vi "Sonar_MLS.vi"() -> ()   [LabVIEW 2016]
uses:
  <vilib>/rvi/Analysis/host/Private/Sample Rate To Loop Time (ticks).vi
  <vilib>/FPGAPlugInAG/sbRIO-9633/niLvFpga_Open_sbRIO-9633.vi
  <vilib>/rvi/interface/common/dynamic/niFpgaDynamicAddResources.vi
  <vilib>/Utility/error.llb/Error Cluster From Error Code.vi
  <vilib>/rvi/errors/niLvFpgaAdjustHostInterfaceError.vi
  <vilib>/FPGAPlugInAG/Dynamic/niLvFpga_Run_Dynamic.vi
  <vilib>/Utility/file.llb/Write Delimited Spreadsheet (string).vi
  <vilib>/FPGAPlugInAG/Dynamic/niLvFpga_Close_Dynamic.vi
  <vilib>/rvi/interface/nirviOpenFPGA/nirviOpenFPGA.xnode
  FPGA Bitfiles/sbRIOtest_FPGATarget2_DAQgenV4_wkZzV3iQ7fI.lvbitx
  DAQgenV4.vi
  <vilib>/rvi/interface/nirviReadWriteControl/nirviReadWriteControl.xnode
  <vilib>/rvi/interface/nirviMethod/nirviMethod.xnode
  <vilib>/rvi/interface/nirviCloseFPGA/nirviCloseFPGA.xnode
  <vilib>/rvi/errors/niLvFpgaMergeErrorWithErrorCode.vi
  <vilib>/rvi/interface/Simulation/niFpgaSimulationCallBeginRW.vi
  <vilib>/FPGAPlugInAG/Dynamic/niLvFpga_StartFifo_Dynamic.vi
  <vilib>/rvi/Analysis/host/Public/NI_FpgaMspHost.lvlib
  NiFpgaLv.dll
  <vilib>/FPGAPlugInAG/Dynamic/niLvFpga_ReadFifo_Dynamic.vi
  <vilib>/FPGAPlugInAG/Dynamic/niLvFpga_WriteFifo_Dynamic.vi
panel:
  out "Fs, out (Hz)":dbl format="%#_6p"
  out "Fs, in (Hz)":dbl
  in  "Iterations":i32=25
  in  "VISA resource name":refnum<visa-resource-name>="ASRL1::INSTR"
  out "?":string
  in  "Interpulse Time (ms)":u32=1300
  out "Aggregate Input Rate (Hz)":dbl
  in  "?":bool
  in  "Chirp Length (ms)":i32=5
  out "Echo":dbl[][](graph)
  in  "Samples to Read":i32=4000
  out "Wave Output":dbl[](graph)=[0.5, 0.5001220703125, 0.50048828125, 0.5010986328125, 0.501953125, 0.5029296875, 0.504150390625, 0.50537109375, 0.5064697265625, 0.50732421875, 0.5078125, 0.50732421875, 0.505859375, 0.5030517578125, 0.4986572265625, 0.4925537109375, 0.48486328125, 0.47607421875, 0.466796875, 0.4583740234375, 0.4522705078125, 0.4501953125, 0.4539794921875, 0.4647216796875, 0.4830322265625, 0.5078125, 0.5364990234375, 0.564697265625, 0.5865478515625, 0.5960693359375, 0.5880126953125, 0.56005859375, 0.51416015625, 0.4578857421875, 0.4039306640625, 0.3671875, 0.362060546875, 0.395751953125, 0.46533203125, 0.55419921875, 0.6357421875, 0.6796875, 0.6634521484375, 0.5838623046875, 0.463134765625, 0.345458984375, 0.2823486328125, 0.309814453125, 0.4273681640625, 0.5899658203125, 0.7216796875, 0.750244140625, 0.647705078125, 0.455810546875, 0.2747802734375, 0.213623046875, 0.32275390625, 0.5509033203125, 0.760986328125, 0.8094482421875, 0.6470947265625, 0.3704833984375, 0.1728515625, 0.2109375, 0.4754638671875, 0.7733154296875, 0.862060546875, 0.650146484375, 0.298583984375, 0.10986328125, 0.26806640625, 0.6494140625, 0.9031982421875, 0.7716064453125, 0.362548828125, 0.0799560546875, 0.2296142578125, 0.675048828125, 0.94189453125, 0.7196044921875, 0.238525390625, 0.0513916015625, 0.3975830078125, 0.877685546875, 0.8968505859375, 0.410400390625, 0.0303955078125, 0.2659912109375, 0.822265625, 0.94384765625, 0.4442138671875, 0.0172119140625, 0.28759765625, 0.8759765625, 0.9034423828125, 0.3118896484375, 0.0091552734375, 0.483642578125, 0.9871826171875, 0.6937255859375, 0.076171875, 0.17529296875, 0.8331298828125, 0.90869140625, 0.259033203125, 0.044921875, 0.663330078125, 0.975830078125, 0.391357421875, 0.0184326171875, 0.5802001953125, 0.979248046875, 0.4212646484375, 0.0286865234375, 0.6031494140625, 0.9560546875, 0.348388671875, 0.072509765625, 0.71923828125, 0.8770751953125, 0.2025146484375, 0.2047119140625, 0.87158203125, 0.6761474609375, 0.0802001953125, 0.477783203125, 0.9163818359375, 0.351318359375, 0.1612548828125, 0.8004150390625, 0.6805419921875, 0.1173095703125, 0.532958984375, 0.8494873046875, 0.2613525390625, 0.312255859375, 0.8492431640625, 0.446044921875, 0.2041015625, 0.7640380859375, 0.5853271484375, 0.1837158203125, 0.6695556640625, 0.660888671875, 0.2047119140625, 0.603271484375, 0.686279296875, 0.2335205078125, 0.573974609375, 0.6785888671875, 0.2564697265625, 0.5772705078125, 0.6473388671875, 0.274658203125, 0.603515625, 0.595458984375, 0.2991943359375, 0.6385498046875, 0.52490234375, 0.344482421875, 0.6614990234375, 0.446533203125, 0.4193115234375, 0.648193359375, 0.385986328125, 0.5128173828125, 0.5849609375, 0.37744140625, 0.587158203125, 0.4908447265625, 0.43603515625, 0.595458984375, 0.42333984375, 0.524658203125, 0.53076171875, 0.435302734375, 0.566650390625, 0.458251953125, 0.5052490234375, 0.52685546875, 0.4564208984375, 0.5426025390625, 0.471923828125, 0.5081787109375, 0.509765625, 0.479248046875, 0.5234375, 0.4805908203125, 0.51171875, 0.4964599609375, 0.4971923828125, 0.50634765625, 0.492919921875, 0.5059814453125, 0.4959716796875, 0.5020751953125, 0.499267578125, 0.5, 0.5001220703125, 0.4998779296875]
  in  "Initial Frequency (Hz)":dbl=20000.0
  in  "Final Frequency (Hz)":dbl=100000.0
  in  "Amplitude":dbl=2.0
  # "Echo-Pulse Sonar V6"
  # "To access the data, go to your web browser and type ftp://169.254.32.143/ni-rt/startup/"
  # "Wave Maker"
  # "Adding:\n-Digital signal trigger outputs to Pi\n-Sending data via serial to the Pi"
  # "Logger"
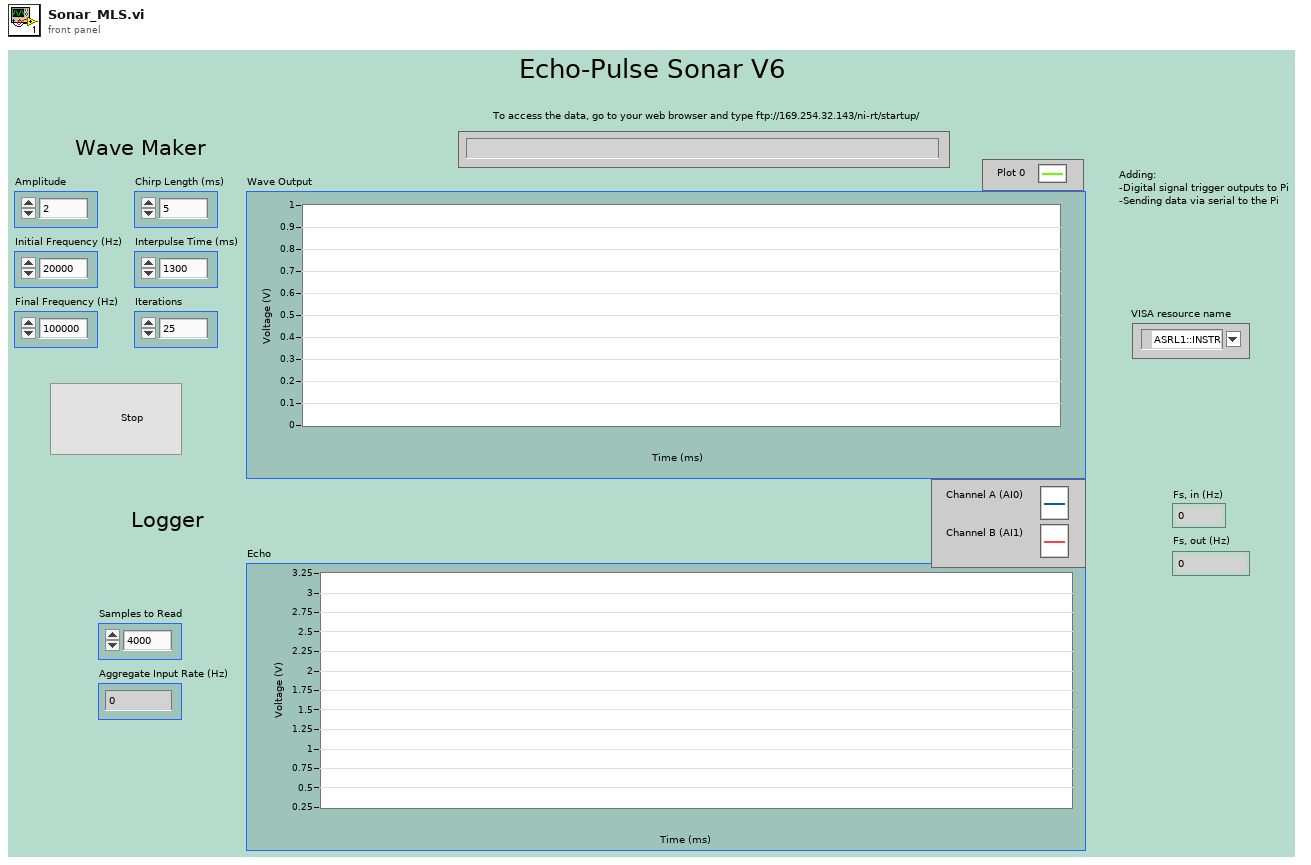
[diagram p1: front panel]
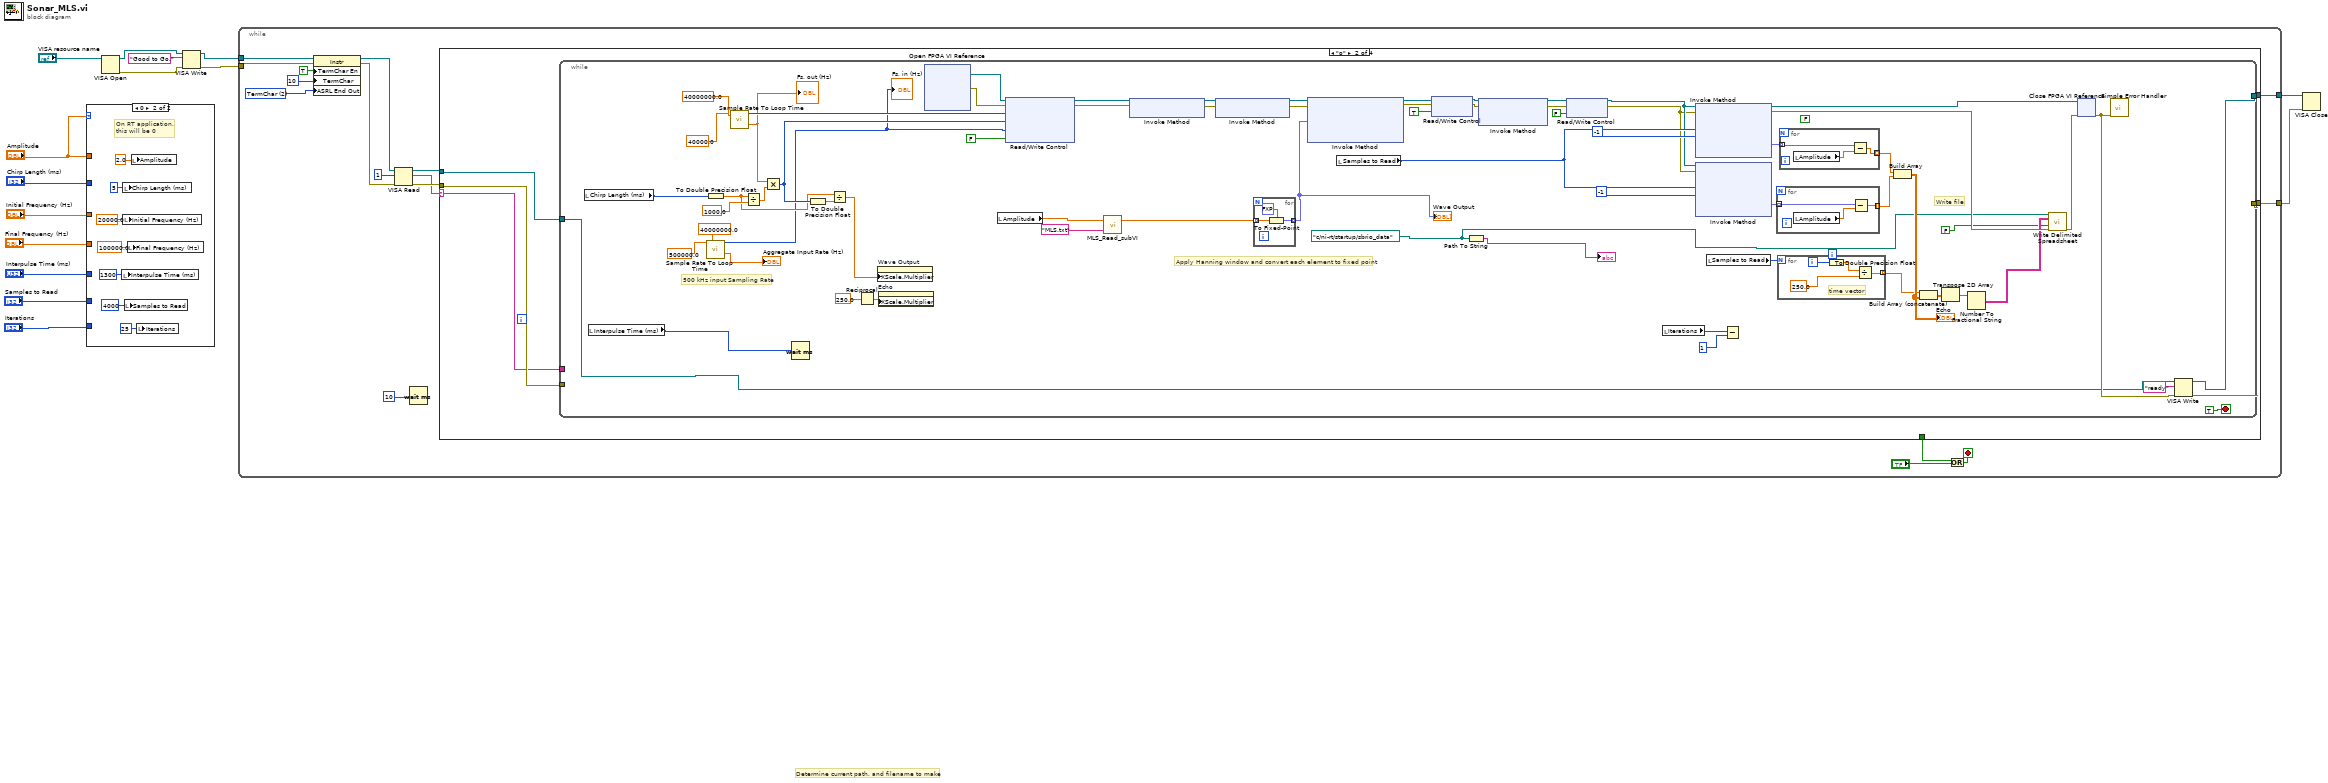
[diagram p0: block diagram]
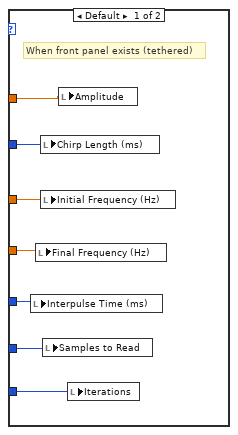
[diagram p2: hidden frame]
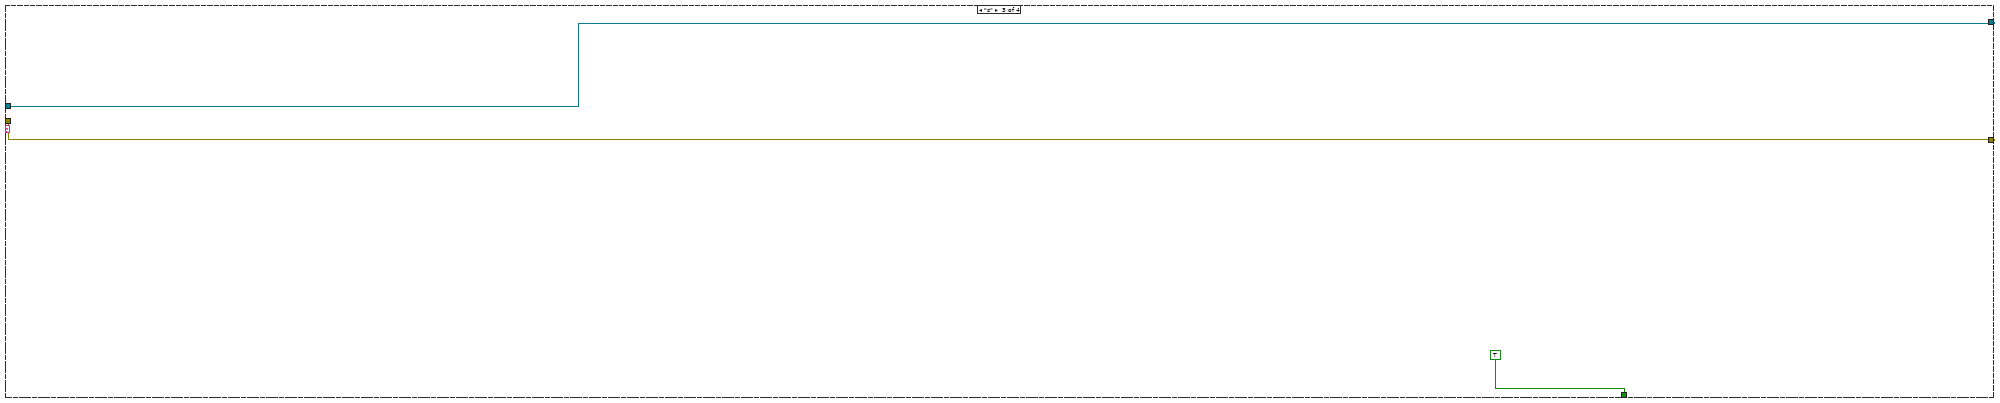
[diagram p4: hidden frame]
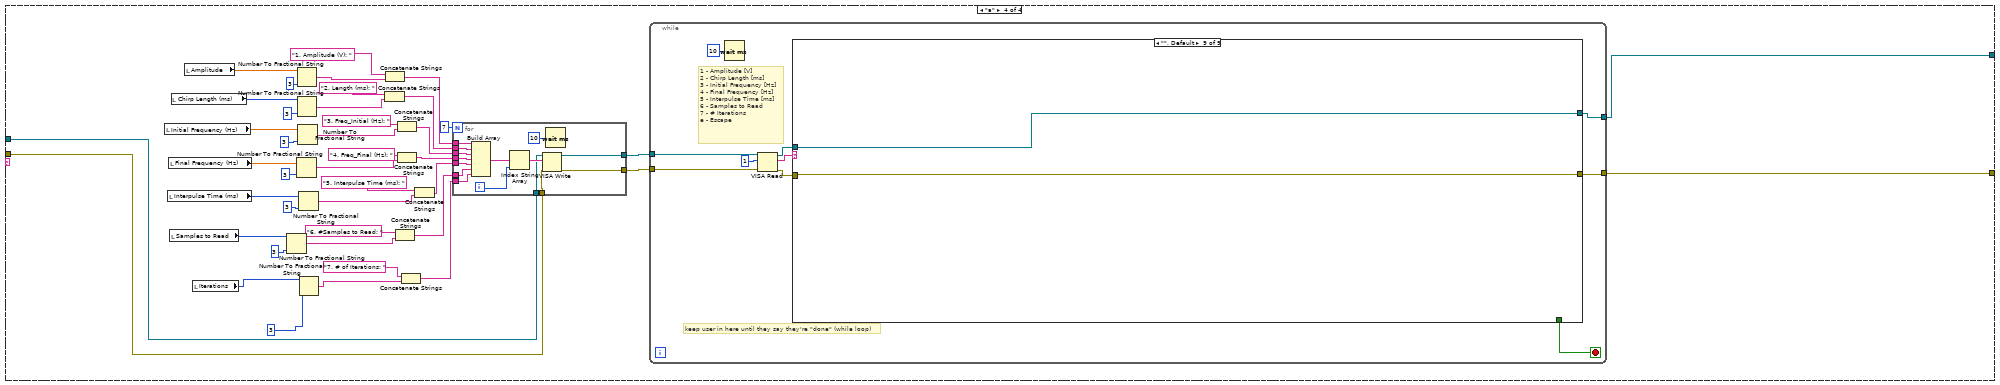
[diagram p5: hidden frame]
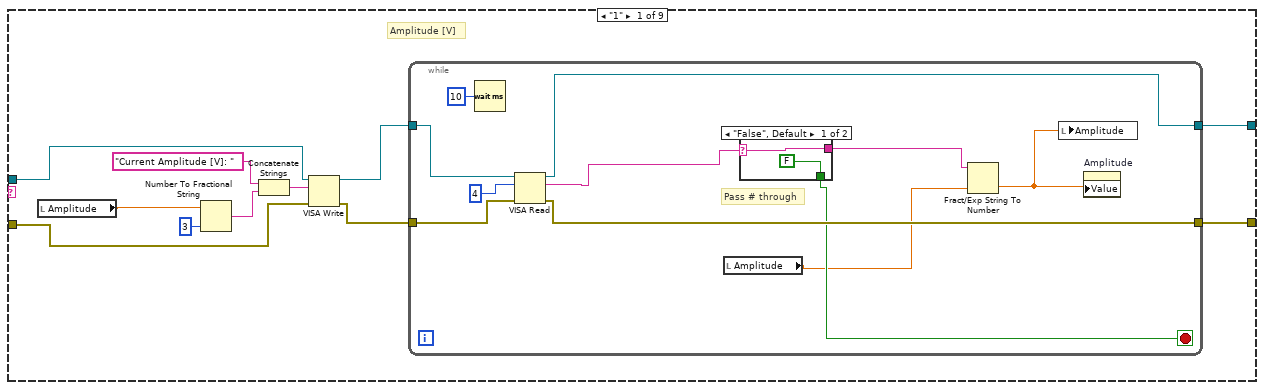
[diagram p6: hidden frame]
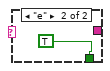
[diagram p7: hidden frame]
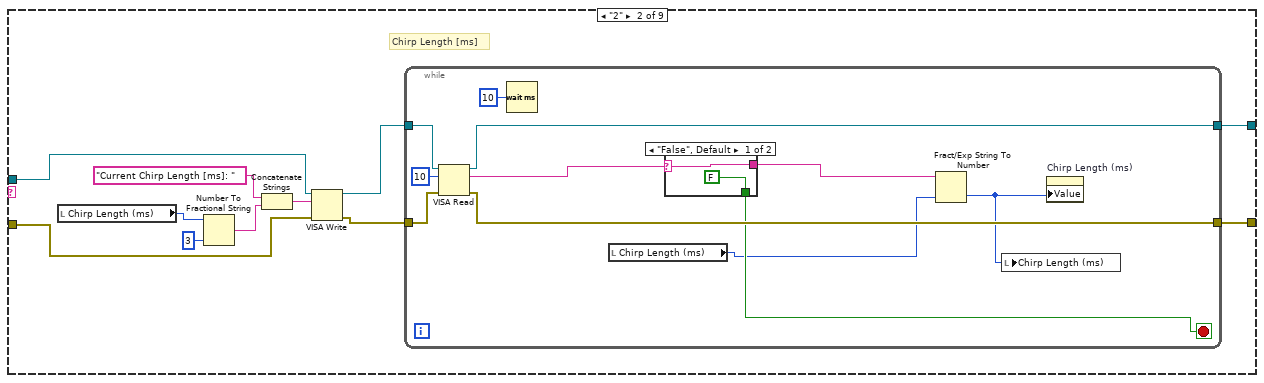
[diagram p8: hidden frame]
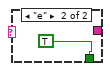
[diagram p9: hidden frame]
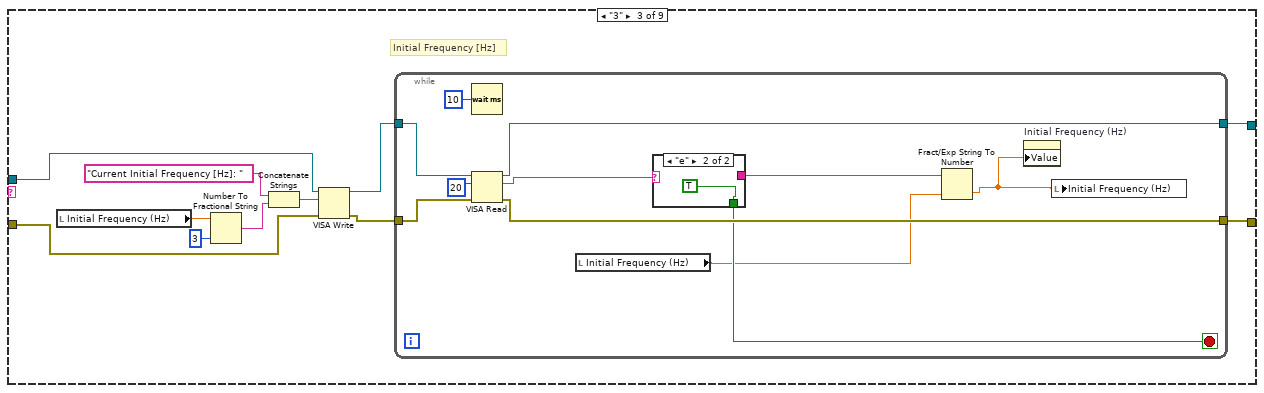
[diagram p10: hidden frame]
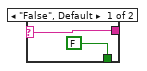
[diagram p11: hidden frame]
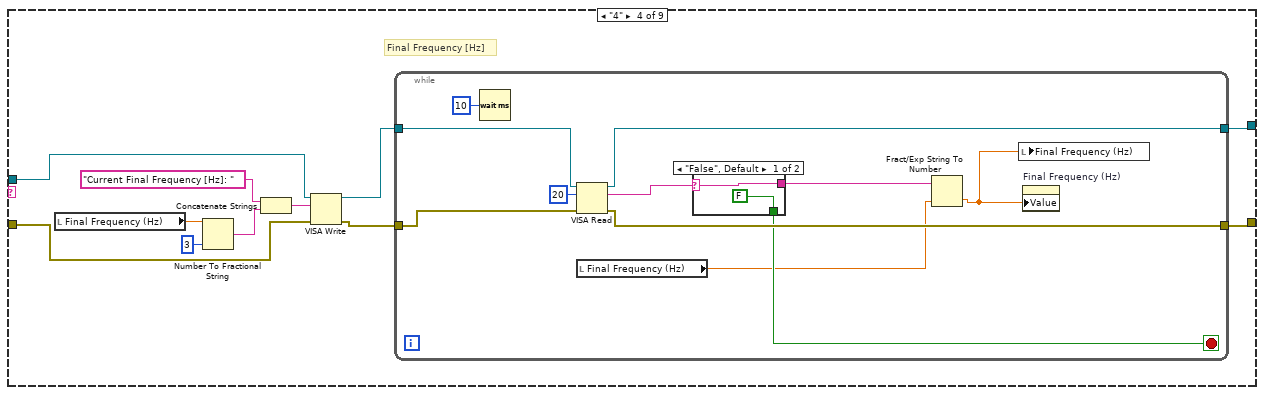
[diagram p12: hidden frame]
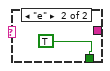
[diagram p13: hidden frame]
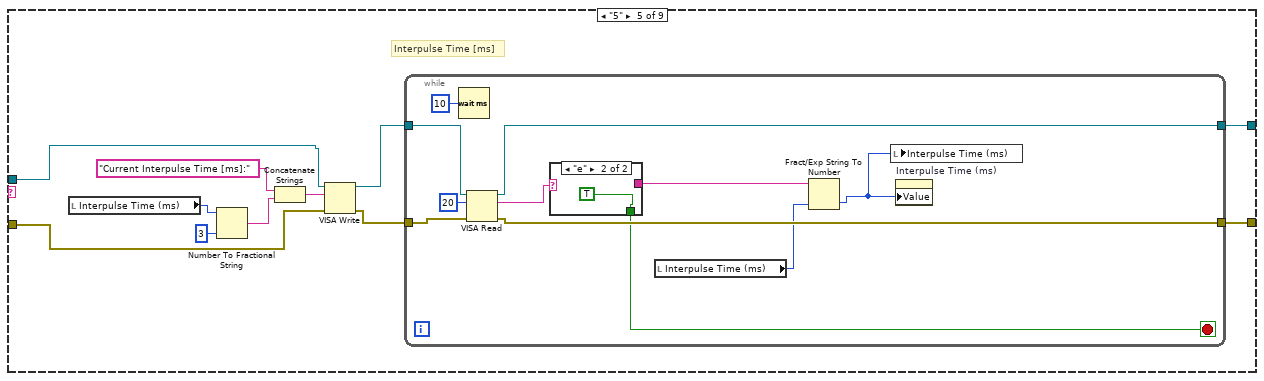
[diagram p14: hidden frame]
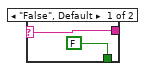
[diagram p15: hidden frame]
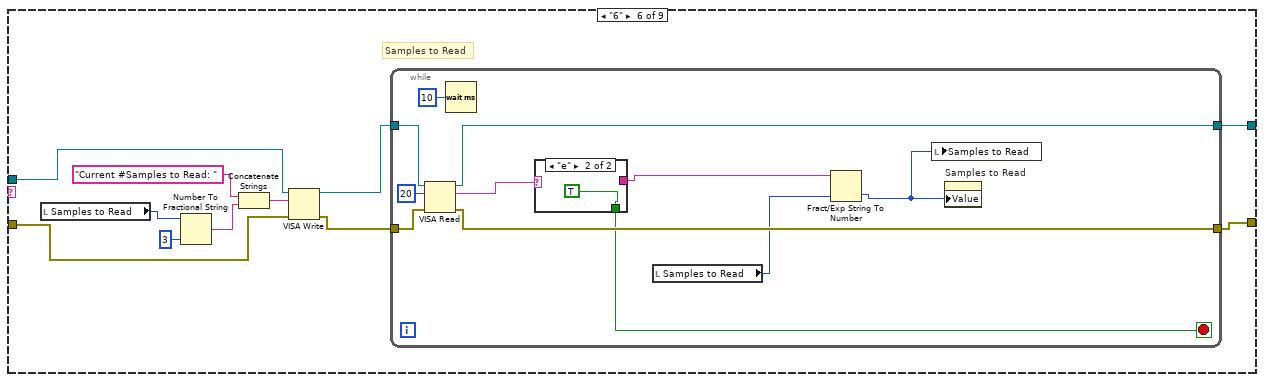
[diagram p16: hidden frame]
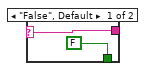
[diagram p17: hidden frame]
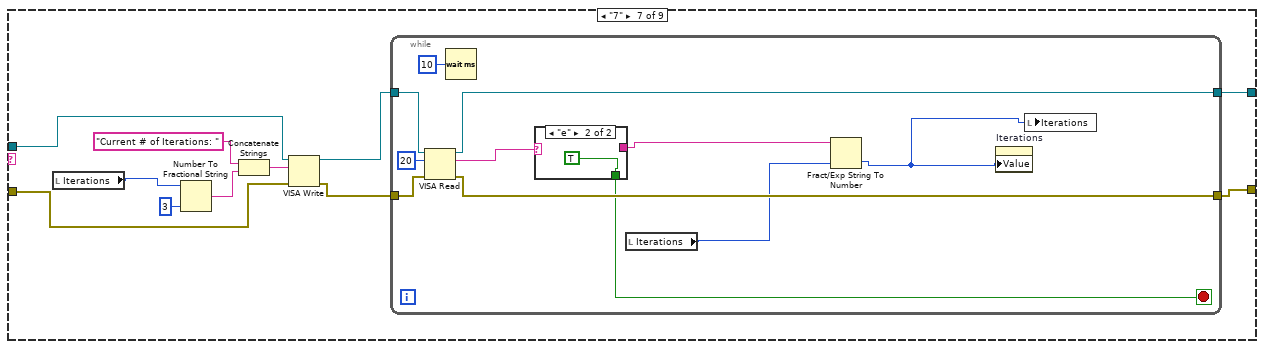
[diagram p18: hidden frame]
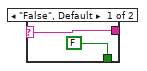
[diagram p19: hidden frame]
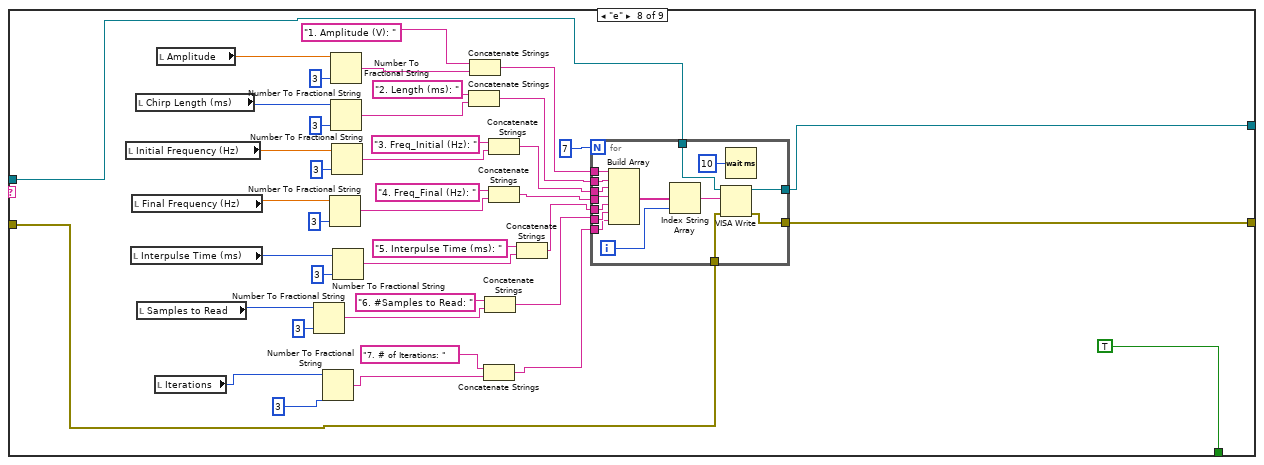
[diagram p20: hidden frame]
diagram:
  # "Determine current path, and filename to make"
  n1 = case shown="0" "Amplitude" {
    tunnel: "Amplitude" -> [w22 _]
    tunnel: "Chirp Length (ms)" -> [w21 _]
    tunnel: "Initial Frequency (Hz)" -> [w20 _]
    tunnel: "Final Frequency (Hz)" -> [w19 _]
    tunnel: "Interpulse Time (ms)" -> [w18 _]
    tunnel: "Samples to Read" -> [w17 _]
    tunnel: "Iterations" -> [w16 _]
    frame Default {
      # "When front panel exists (tethered)"
      n2 = local write "Interpulse Time (ms)"(w18) -> ()
      n3 = local write "Final Frequency (Hz)"(w19) -> ()
      n4 = local write "Chirp Length (ms)"(w21) -> ()
      n5 = local write "Initial Frequency (Hz)"(w20) -> ()
      n6 = local write "Samples to Read"(w17) -> ()
      n7 = local write "Amplitude"(w22) -> ()
      n8 = local write "Iterations"(w16) -> ()
    }
    frame 0 {
      # "On RT application,\nthis will be 0"
      n9 = local write "Interpulse Time (ms)"(u32 1300 ("Interpulse Time (ms)")) -> ()
      n10 = local write "Chirp Length (ms)"(5 ("Chirp Length (ms)")) -> ()
      n11 = local write "Initial Frequency (Hz)"(20000.0 ("Initial Frequency (Hz)")) -> ()
      n12 = local write "Samples to Read"(4000 ("Samples to Read")) -> ()
      n13 = local write "Final Frequency (Hz)"(100000.0 ("Final Frequency (Hz)")) -> ()
      n14 = local write "Amplitude"(2.0 ("Amplitude")) -> ()
      n15 = local write "Iterations"(25 ("Iterations")) -> ()
    }
  }
  n16 = VISA Open(VISA resource name="VISA resource name") -> (VISA resource name=w12:refnum<visa-resource-name>, error out=w11:errorcluster)  [unwired: 4 in]
  n17 = VISA Write(VISA resource name=w12, write buffer="Good to Go.", error in (no error)=w11) -> (VISA resource name out=w9:refnum<visa-resource-name>, error out=w8:errorcluster)  [unwired: 1 out]
  n18 = while {
    tunnel: [w43] -> w14
    tunnel: [w42] -> w13
    tunnel: w9 -> [w33]
    tunnel: w8 -> [w32]
    stop <- w39 stop-if-true
    w34 = u16 2 items=["None", "Last Bit", "TermChar", "Break"] ("Serial Settings:End Mode for Writes")
    n19 = property class="Instr"(reference=w33, error in=w32, "TermChar En"=TRUE ("Message Based Settings:Termination Character Enable"), "TermChar"=u8 10 ("Message Based Settings:Termination Character"), "ASRL End Out"=w34) -> (reference out=w37:refnum<visa-resource-name>, error out=w38:errorcluster)
    n20 = VISA Read(VISA resource name=w37, byte count=u32 1, error in (no error)=w38) -> (VISA resource name out=w45:refnum<visa-resource-name>, read buffer=w40:string, error out=w44:errorcluster)  [unwired: 1 out]
    n21 = Wait (ms)(milliseconds to wait=u32 10) -> ()  [unwired: 1 out]
    n22 = case shown="\"o\"" w40 {
      selector: w40 -> [_ w51 _ _]
      tunnel: w45 -> [w48 w53 w136 w160]
      tunnel: w44 -> [w47 w52 w135 w159]
      tunnel: [w48 w50 w136 w150] -> w43
      tunnel: [w47 w49 w135 w149] -> w42
      tunnel: [_ _ TRUE _] -> w30
      frame "False", Default {
      }
      frame "o" {
        n23 = while {
          tunnel: w53 -> [w65]
          tunnel: w52 -> [_]
          tunnel: w51 -> [_]
          tunnel: [w121] -> w50
          tunnel: [w59] -> w49
          stop <- TRUE stop-if-true
          w60 = path "c:/ni-rt/startup/sbrio_data"
          (unwired) FALSE ("Wavegen!")
          # "Write file"
          # "Apply Hanning window and convert each element to fixed point"
          # "500 kHz input Sampling Rate"
          n24 = local read "Chirp Length (ms)"() -> (w73:i32)
          n25 = local read "Interpulse Time (ms)"() -> (w69:u32)
          n26 = call-poly <vilib>:"Sample Rate To Loop Time.vi"("sample rate (S/s)"=500000.0, "FPGA clock rate (Hz)"=40000000.0) -> ("count (ticks/S)"=w68:u32, "actual sample rate (S/s)"=→"Aggregate Input Rate (Hz)":dbl)  [unwired: 11 in, 1 out]
          "Fs, in (Hz)" <- w68
          n27 = To Double Precision Float(number=w73) -> (double precision float=w86:dbl)
          n28 = call-poly <vilib>:"Sample Rate To Loop Time.vi"("sample rate (S/s)"=40000.0, "FPGA clock rate (Hz)"=40000000.0) -> ("count (ticks/S)"=w107:u32, "actual sample rate (S/s)"=w89:dbl)  [unwired: 11 in, 1 out]
          "Fs, out (Hz)" <- w89
          n29 = Divide(x=w86, y=1000.0) -> (x/y=w87:dbl)
          n30 = Multiply(x=w89, y=w87) -> (x*y=w99:i16)
          n31 = Wait (ms)(milliseconds to wait=w69) -> ()  [unwired: 1 out]
          n32 = To Double Precision Float(number=w99) -> (double precision float=w116:dbl)
          n33 = Divide(x=w86, y=w116) -> (x/y=w90:dbl)
          n34 = Reciprocal(x=250.0) -> (1/x=w100:dbl)
          n35 = property on="Wave Output" class="WFGraph (strict)"("XScale.Multiplier"=w90) -> ()  [unwired: 2 in, 2 out]
          n36 = property on="Echo" class="WFGraph (strict)"("XScale.Multiplier"=w100) -> ()  [unwired: 2 in, 2 out]
          n37 = xnode "Open FPGA VI Reference"() -> ("FPGA VI Reference Out"=w92:refnum<k20>, "error out"=w91:errorcluster)  [unwired: 2 in]
          n38 = local read "Amplitude"() -> (w55:dbl)
          n39 = xnode "Read/Write Control"("FPGA VI Reference In"=w92, "error in"=w91, "Sampling Rate (Hz)"=w107, "# Samples"=w99, "Count(Ticks)"=w68, "Wavegen!"=FALSE) -> ("FPGA VI Reference Out"=w94:refnum<k20>, "error out"=w93:errorcluster)
          n40 = call "MLS_Read_subVI.vi"("Filename"="MLS.txt", "Amplitude"=w55) -> ("Waveform Graph"=w54:dbl[])  [unwired: 1 out]
          n41 = xnode "Invoke Method"("FPGA VI Reference In"=w94, "error in"=w93) -> ("FPGA VI Reference Out"=w96:refnum<k20>, "error out"=w95:errorcluster)
          n42 = xnode "Invoke Method"("FPGA VI Reference In"=w96, "error in"=w95) -> ("FPGA VI Reference Out"=w98:refnum<k20>, "error out"=w97:errorcluster)
          n43 = for {
            tunnel: [w133] -> w115 mode=indexing
            tunnel: w54 -> [w132] mode=indexing
            n44 = To Fixed-Point(fixed-point type=fxp<+,16,3> 0.0 ("AO0"), number=w132) -> (fixed-point=w133:fxp<+,16,3>)
          }
          "Wave Output" <- w115
          n45 = xnode "Invoke Method"("FPGA VI Reference In"=w98, "error in"=w97, "Data"=w115) -> ("FPGA VI Reference Out"=w106:refnum<k20>, "error out"=w105:errorcluster)  [unwired: 1 in, 1 out]
          n46 = local read "Samples to Read"() -> (w72:i32)
          n47 = xnode "Read/Write Control"("FPGA VI Reference In"=w106, "error in"=w105, "Wavegen!"=TRUE) -> ("FPGA VI Reference Out"=w104:refnum<k20>, "error out"=w103:errorcluster)
          n48 = Path To String(path=w60) -> (string=→"?":string)
          n49 = xnode "Invoke Method"("FPGA VI Reference In"=w104, "error in"=w103) -> ("FPGA VI Reference Out"=w63:refnum<k20>, "error out"=w62:errorcluster)  [unwired: 1 in]
          n50 = xnode "Read/Write Control"("FPGA VI Reference In"=w63, "error in"=w62, "Wavegen!"=FALSE) -> ("FPGA VI Reference Out"=w58:refnum<k20>, "error out"=w57:errorcluster)
          n51 = local read "Iterations"() -> (w71:i32)
          n52 = xnode "Invoke Method"("FPGA VI Reference In"=w58, "error in"=w57, "Number of Elements"=w72, "Timeout (ms)"=-1) -> ("FPGA VI Reference Out"=w109:refnum<k20>, "error out"=w85:errorcluster, "Data"=w111:fxp<+,16,3>[])  [unwired: 1 out]
          n53 = xnode "Invoke Method"("FPGA VI Reference In"=w58, "error in"=w57, "Number of Elements"=w72, "Timeout (ms)"=-1) -> ("Data"=w110:fxp<+,16,3>[])  [unwired: 3 out]
          n54 = local read "Samples to Read"() -> (w83:i32)
          n55 = Subtract(x=w71, y=1) -> ()  [unwired: 1 out]
          n56 = for {
            tunnel: w110 -> [w131] mode=indexing
            tunnel: [w129] -> w77 mode=indexing
            n57 = local read "Amplitude"() -> (w130:dbl)
            n58 = Subtract(x=w131, y=w130) -> (x-y=w129:dbl)
          }
          n59 = for {
            N: w83 -> [_]
            tunnel: [w123] -> w79 mode=indexing
            i -> [w125]
            # "time vector"
            n60 = To Double Precision Float(number=w125) -> (double precision float=w124:dbl)
            n61 = Divide(x=w124, y=250.0) -> (x/y=w123:dbl)
          }
          n62 = for {
            tunnel: w111 -> [w128] mode=indexing
            tunnel: [w126] -> w78 mode=indexing
            n63 = local read "Amplitude"() -> (w127:dbl)
            n64 = Subtract(x=w128, y=w127) -> (x-y=w126:dbl)
          }
          n65 = Build Array(w78, w77) -> (w82:dbl[][])
          "Echo" <- w82
          n66 = Build Array (concatenate)(w79, w82) -> (w81:dbl[][])
          n67 = Transpose 2D Array(2D array=w81) -> (transposed array=w80:dbl[][])
          n68 = Number To Fractional String(number=w80) -> (F-format string=w67:string[][])  [unwired: 3 in]
          n69 = call-poly <vilib>:"Write Delimited Spreadsheet.vi"("file path (dialog if empty)"=w60, "2D data"=w67, "append to file? (new file:F)"=FALSE, "error in (no error)"=w85) -> ("error out"=w84:errorcluster)  [unwired: 10 in, 1 out]
          n70 = xnode "Close FPGA VI Reference"("FPGA VI Reference In"=w109, "error in"=w84) -> ("error out"=w74:errorcluster)
          n71 = call <vilib>:"Simple Error Handler.vi"("error in (no error)"=w74) -> ()  [unwired: 4 in, 5 out]
          n72 = VISA Write(VISA resource name=w65, write buffer="ready", error in (no error)=w74) -> (VISA resource name out=w121:refnum<visa-resource-name>, error out=w59:errorcluster)  [unwired: 1 out]
        }
      }
      frame "s" {
      }
      frame "a" {
        n73 = local read "Initial Frequency (Hz)"() -> (w146:dbl)
        n74 = local read "Interpulse Time (ms)"() -> (w148:u32)
        n75 = local read "Final Frequency (Hz)"() -> (w147:dbl)
        n76 = local read "Samples to Read"() -> (w143:i32)
        n77 = local read "Chirp Length (ms)"() -> (w145:i32)
        n78 = local read "Amplitude"() -> (w144:dbl)
        n79 = local read "Iterations"() -> (w141:i32)
        n80 = Number To Fractional String(number=w143, precision (6)=i16 3) -> (F-format string=w168:string)  [unwired: 2 in]
        n81 = Number To Fractional String(number=w147, precision (6)=i16 3) -> (F-format string=w170:string)  [unwired: 2 in]
        n82 = Number To Fractional String(number=w144, precision (6)=i16 3) -> (F-format string=w178:string)  [unwired: 2 in]
        n83 = Number To Fractional String(number=w145, precision (6)=i16 3) -> (F-format string=w172:string)  [unwired: 2 in]
        n84 = Number To Fractional String(number=w146, precision (6)=i16 3) -> (F-format string=w171:string)  [unwired: 2 in]
        n85 = Number To Fractional String(number=w148, precision (6)=i16 3) -> (F-format string=w169:string)  [unwired: 2 in]
        n86 = Number To Fractional String(number=w141, precision (6)=i16 3) -> (F-format string=w140:string)  [unwired: 2 in]
        n87 = Concatenate Strings("2. Length (ms): " ("string"), w172) -> (w167:string)
        n88 = Concatenate Strings("1. Amplitude (V): " ("string"), w178) -> (w153:string)
        n89 = Concatenate Strings("6. #Samples to Read: " ("string"), w168) -> (w163:string)
        n90 = Concatenate Strings("3. Freq_Initial (Hz): " ("string"), w171) -> (w166:string)
        n91 = Concatenate Strings("4. Freq_Final (Hz): " ("string"), w170) -> (w165:string)
        n92 = Concatenate Strings("7. # of Iterations: " ("string"), w140) -> (w138:string)
        n93 = Concatenate Strings("5. Interpulse Time (ms): " ("string"), w169) -> (w164:string)
        n94 = for {
          N: 7 -> [_]
          tunnel: w167 -> [w437]
          tunnel: w166 -> [w436]
          tunnel: w165 -> [w435]
          tunnel: w164 -> [w434]
          tunnel: w163 -> [w424]
          tunnel: w160 -> [w430]
          tunnel: w159 -> [w429]
          tunnel: [w428] -> w162
          tunnel: [w427] -> w161
          tunnel: w153 -> [w426]
          tunnel: w138 -> [w423]
          i -> [w432]
          n95 = Build Array(w426, w437, w436, w435, w434, w424, w423) -> (w433:string[])
          n96 = Index String Array(1:w432, 2:w433) -> (0:w431:string)  [unwired: 1 in]
          n97 = VISA Write(VISA resource name=w430, write buffer=w431, error in (no error)=w429) -> (VISA resource name out=w428:refnum<visa-resource-name>, error out=w427:errorcluster)  [unwired: 1 out]
          n98 = Wait (ms)(milliseconds to wait=u32 10) -> ()  [unwired: 1 out]
        }
        n99 = while {
          tunnel: w162 -> [w189]
          tunnel: w161 -> [w188]
          tunnel: [w183] -> w150
          tunnel: [w184] -> w149
          stop <- w187 stop-if-true
          # "1 - Amplitude [V]\n2 - Chirp Length [ms]\n3 - Initial Frequency [Hz]\n4 - Final Frequency [Hz]\n5 - Interpulse Time [ms]\n6 - Samples to Read\n7 - # Iterations\ne - Escape"
          # "keep user in here until they say they're \"done\" (while loop)"
          n100 = Wait (ms)(milliseconds to wait=u32 10) -> ()  [unwired: 1 out]
          n101 = VISA Read(VISA resource name=w189, byte count=u32 1, error in (no error)=w188) -> (VISA resource name out=w182:refnum<visa-resource-name>, read buffer=w181:string, error out=w180:errorcluster)  [unwired: 1 out]
          n102 = case shown="\"\", Default" w181 {
            tunnel: [_ _ _ _ _ _ _ TRUE _] -> w187
            tunnel: w182 -> [w193 w219 w244 w269 w294 w319 w344 w379 w422]
            tunnel: w180 -> [w194 w218 w243 w268 w293 w318 w343 w378 w421]
            tunnel: [w200 w225 w250 w275 w300 w325 w350 w377 w422] -> w183
            tunnel: [w199 w224 w249 w274 w299 w324 w349 w376 w421] -> w184
            frame "1" {
              # "Amplitude [V]"
              n103 = local read "Amplitude"() -> (w190:dbl)
              n104 = Number To Fractional String(number=w190, precision (6)=i16 3) -> (F-format string=w195:string)  [unwired: 2 in]
              n105 = Concatenate Strings("Current Amplitude [V]: " ("string"), w195) -> (w198:string)
              n106 = VISA Write(VISA resource name=w193, write buffer=w198, error in (no error)=w194) -> (VISA resource name out=w192:refnum<visa-resource-name>, error out=w191:errorcluster)  [unwired: 1 out]
              n107 = while {
                tunnel: w192 -> [w211]
                tunnel: [w205] -> w200
                tunnel: w191 -> [w210]
                tunnel: [w209] -> w199
                stop <- w204 stop-if-true
                # "Pass # through"
                n108 = Wait (ms)(milliseconds to wait=u32 10) -> ()  [unwired: 1 out]
                n109 = VISA Read(VISA resource name=w211, byte count=u32 4, error in (no error)=w210) -> (VISA resource name out=w205:refnum<visa-resource-name>, read buffer=w206:string, error out=w209:errorcluster)  [unwired: 1 out]
                n110 = local read "Amplitude"() -> (w201:dbl)
                n111 = case shown="\"False\", Default" w206 {
                  selector: w206 -> [w213 _]
                  tunnel: [FALSE TRUE] -> w204
                  tunnel: [w213 _] -> w203
                  frame "False", Default {
                  }
                  frame "e" {
                  }
                }
                n112 = Fract/Exp String To Number(string=w203, default (0 dbl)=w201) -> (number=w202:dbl)  [unwired: 2 in, 1 out]
                n113 = local write "Amplitude"(w202) -> ()
                n114 = property on="Amplitude" class="DigNum (strict)"("Value"=w202) -> ()  [unwired: 2 in, 2 out]
              }
            }
            frame "2" {
              # "Chirp Length [ms]"
              n115 = local read "Chirp Length (ms)"() -> (w215:i32)
              n116 = Number To Fractional String(number=w215, precision (6)=i16 3) -> (F-format string=w220:string)  [unwired: 2 in]
              n117 = Concatenate Strings("Current Chirp Length [ms]: " ("string"), w220) -> (w223:string)
              n118 = VISA Write(VISA resource name=w219, write buffer=w223, error in (no error)=w218) -> (VISA resource name out=w217:refnum<visa-resource-name>, error out=w216:errorcluster)  [unwired: 1 out]
              n119 = while {
                tunnel: w217 -> [w236]
                tunnel: [w234] -> w225
                tunnel: w216 -> [w235]
                tunnel: [w233] -> w224
                stop <- w229 stop-if-true
                n120 = VISA Read(VISA resource name=w236, byte count=u32 10, error in (no error)=w235) -> (VISA resource name out=w234:refnum<visa-resource-name>, read buffer=w231:string, error out=w233:errorcluster)  [unwired: 1 out]
                n121 = Wait (ms)(milliseconds to wait=u32 10) -> ()  [unwired: 1 out]
                n122 = local read "Chirp Length (ms)"() -> (w226:i32)
                n123 = case shown="\"False\", Default" w231 {
                  selector: w231 -> [w238 _]
                  tunnel: [FALSE TRUE] -> w229
                  tunnel: [w238 _] -> w230
                  frame "False", Default {
                  }
                  frame "e" {
                  }
                }
                n124 = Fract/Exp String To Number(string=w230, default (0 dbl)=w226) -> (number=w227:i32)  [unwired: 2 in, 1 out]
                n125 = local write "Chirp Length (ms)"(w227) -> ()
                n126 = property on="Chirp Length (ms)" class="DigNum (strict)"("Value"=w227) -> ()  [unwired: 2 in, 2 out]
              }
            }
            frame "3" {
              # "Initial Frequency [Hz]"
              n127 = local read "Initial Frequency (Hz)"() -> (w240:dbl)
              n128 = Number To Fractional String(number=w240, precision (6)=i16 3) -> (F-format string=w245:string)  [unwired: 2 in]
              n129 = Concatenate Strings("Current Initial Frequency [Hz]: " ("string"), w245) -> (w248:string)
              n130 = VISA Write(VISA resource name=w244, write buffer=w248, error in (no error)=w243) -> (VISA resource name out=w242:refnum<visa-resource-name>, error out=w241:errorcluster)  [unwired: 1 out]
              n131 = while {
                tunnel: w242 -> [w261]
                tunnel: [w259] -> w250
                tunnel: w241 -> [w260]
                tunnel: [w258] -> w249
                stop <- w254 stop-if-true
                n132 = Wait (ms)(milliseconds to wait=u32 10) -> ()  [unwired: 1 out]
                n133 = VISA Read(VISA resource name=w261, byte count=u32 20, error in (no error)=w260) -> (VISA resource name out=w259:refnum<visa-resource-name>, read buffer=w256:string, error out=w258:errorcluster)  [unwired: 1 out]
                n134 = local read "Initial Frequency (Hz)"() -> (w252:dbl)
                n135 = case shown="\"e\"" w256 {
                  selector: w256 -> [w263 _]
                  tunnel: [FALSE TRUE] -> w254
                  tunnel: [w263 _] -> w255
                  frame "False", Default {
                  }
                  frame "e" {
                  }
                }
                n136 = Fract/Exp String To Number(string=w255, default (0 dbl)=w252) -> (number=w251:dbl)  [unwired: 2 in, 1 out]
                n137 = property on="Initial Frequency (Hz)" class="DigNum (strict)"("Value"=w251) -> ()  [unwired: 2 in, 2 out]
                n138 = local write "Initial Frequency (Hz)"(w251) -> ()
              }
            }
            frame "4" {
              # "Final Frequency [Hz]"
              n139 = local read "Final Frequency (Hz)"() -> (w265:dbl)
              n140 = Number To Fractional String(number=w265, precision (6)=i16 3) -> (F-format string=w270:string)  [unwired: 2 in]
              n141 = Concatenate Strings("Current Final Frequency [Hz]: " ("string"), w270) -> (w273:string)
              n142 = VISA Write(VISA resource name=w269, write buffer=w273, error in (no error)=w268) -> (VISA resource name out=w267:refnum<visa-resource-name>, error out=w266:errorcluster)  [unwired: 1 out]
              n143 = while {
                tunnel: w267 -> [w286]
                tunnel: [w284] -> w275
                tunnel: w266 -> [w285]
                tunnel: [w283] -> w274
                stop <- w279 stop-if-true
                n144 = Wait (ms)(milliseconds to wait=u32 10) -> ()  [unwired: 1 out]
                n145 = VISA Read(VISA resource name=w286, byte count=u32 20, error in (no error)=w285) -> (VISA resource name out=w284:refnum<visa-resource-name>, read buffer=w281:string, error out=w283:errorcluster)  [unwired: 1 out]
                n146 = local read "Final Frequency (Hz)"() -> (w277:dbl)
                n147 = case shown="\"False\", Default" w281 {
                  selector: w281 -> [w288 _]
                  tunnel: [FALSE TRUE] -> w279
                  tunnel: [w288 _] -> w280
                  frame "False", Default {
                  }
                  frame "e" {
                  }
                }
                n148 = Fract/Exp String To Number(string=w280, default (0 dbl)=w277) -> (number=w276:dbl)  [unwired: 2 in, 1 out]
                n149 = local write "Final Frequency (Hz)"(w276) -> ()
                n150 = property on="Final Frequency (Hz)" class="DigNum (strict)"("Value"=w276) -> ()  [unwired: 2 in, 2 out]
              }
            }
            frame "5" {
              # "Interpulse Time [ms]"
              n151 = local read "Interpulse Time (ms)"() -> (w290:u32)
              n152 = Number To Fractional String(number=w290, precision (6)=i16 3) -> (F-format string=w295:string)  [unwired: 2 in]
              n153 = Concatenate Strings("Current Interpulse Time [ms]:" ("string"), w295) -> (w298:string)
              n154 = VISA Write(VISA resource name=w294, write buffer=w298, error in (no error)=w293) -> (VISA resource name out=w292:refnum<visa-resource-name>, error out=w291:errorcluster)  [unwired: 1 out]
              n155 = while {
                tunnel: w292 -> [w311]
                tunnel: [w309] -> w300
                tunnel: w291 -> [w310]
                tunnel: [w308] -> w299
                stop <- w304 stop-if-true
                n156 = Wait (ms)(milliseconds to wait=u32 10) -> ()  [unwired: 1 out]
                n157 = VISA Read(VISA resource name=w311, byte count=u32 20, error in (no error)=w310) -> (VISA resource name out=w309:refnum<visa-resource-name>, read buffer=w306:string, error out=w308:errorcluster)  [unwired: 1 out]
                n158 = case shown="\"e\"" w306 {
                  selector: w306 -> [w313 _]
                  tunnel: [FALSE TRUE] -> w304
                  tunnel: [w313 _] -> w305
                  frame "False", Default {
                  }
                  frame "e" {
                  }
                }
                n159 = local read "Interpulse Time (ms)"() -> (w301:u32)
                n160 = Fract/Exp String To Number(string=w305, default (0 dbl)=w301) -> (number=w302:u32)  [unwired: 2 in, 1 out]
                n161 = local write "Interpulse Time (ms)"(w302) -> ()
                n162 = property on="Interpulse Time (ms)" class="DigNum (strict)"("Value"=w302) -> ()  [unwired: 2 in, 2 out]
              }
            }
            frame "6" {
              # "Samples to Read"
              n163 = local read "Samples to Read"() -> (w315:i32)
              n164 = Number To Fractional String(number=w315, precision (6)=i16 3) -> (F-format string=w320:string)  [unwired: 2 in]
              n165 = Concatenate Strings("Current #Samples to Read: " ("string"), w320) -> (w323:string)
              n166 = VISA Write(VISA resource name=w319, write buffer=w323, error in (no error)=w318) -> (VISA resource name out=w317:refnum<visa-resource-name>, error out=w316:errorcluster)  [unwired: 1 out]
              n167 = while {
                tunnel: w317 -> [w336]
                tunnel: [w334] -> w325
                tunnel: w316 -> [w335]
                tunnel: [w333] -> w324
                stop <- w328 stop-if-true
                n168 = VISA Read(VISA resource name=w336, byte count=u32 20, error in (no error)=w335) -> (VISA resource name out=w334:refnum<visa-resource-name>, read buffer=w331:string, error out=w333:errorcluster)  [unwired: 1 out]
                n169 = Wait (ms)(milliseconds to wait=u32 10) -> ()  [unwired: 1 out]
                n170 = case shown="\"e\"" w331 {
                  selector: w331 -> [w338 _]
                  tunnel: [FALSE TRUE] -> w328
                  tunnel: [w338 _] -> w330
                  frame "False", Default {
                  }
                  frame "e" {
                  }
                }
                n171 = local read "Samples to Read"() -> (w326:i32)
                n172 = Fract/Exp String To Number(string=w330, default (0 dbl)=w326) -> (number=w327:i32)  [unwired: 2 in, 1 out]
                n173 = local write "Samples to Read"(w327) -> ()
                n174 = property on="Samples to Read" class="DigNum (strict)"("Value"=w327) -> ()  [unwired: 2 in, 2 out]
              }
            }
            frame "7" {
              n175 = local read "Iterations"() -> (w340:i32)
              n176 = Number To Fractional String(number=w340, precision (6)=i16 3) -> (F-format string=w345:string)  [unwired: 2 in]
              n177 = Concatenate Strings("Current # of Iterations: " ("string"), w345) -> (w348:string)
              n178 = VISA Write(VISA resource name=w344, write buffer=w348, error in (no error)=w343) -> (VISA resource name out=w342:refnum<visa-resource-name>, error out=w341:errorcluster)  [unwired: 1 out]
              n179 = while {
                tunnel: w342 -> [w361]
                tunnel: [w359] -> w350
                tunnel: w341 -> [w360]
                tunnel: [w358] -> w349
                stop <- w353 stop-if-true
                n180 = VISA Read(VISA resource name=w361, byte count=u32 20, error in (no error)=w360) -> (VISA resource name out=w359:refnum<visa-resource-name>, read buffer=w356:string, error out=w358:errorcluster)  [unwired: 1 out]
                n181 = Wait (ms)(milliseconds to wait=u32 10) -> ()  [unwired: 1 out]
                n182 = case shown="\"e\"" w356 {
                  selector: w356 -> [w363 _]
                  tunnel: [FALSE TRUE] -> w353
                  tunnel: [w363 _] -> w355
                  frame "False", Default {
                  }
                  frame "e" {
                  }
                }
                n183 = local read "Iterations"() -> (w352:i32)
                n184 = Fract/Exp String To Number(string=w355, default (0 dbl)=w352) -> (number=w351:i32)  [unwired: 2 in, 1 out]
                n185 = property on="Iterations" class="DigNum (strict)"("Value"=w351) -> ()  [unwired: 2 in, 2 out]
                n186 = local write "Iterations"(w351) -> ()
              }
            }
            frame "e" {
              n187 = local read "Initial Frequency (Hz)"() -> (w373:dbl)
              n188 = local read "Interpulse Time (ms)"() -> (w371:u32)
              n189 = local read "Final Frequency (Hz)"() -> (w372:dbl)
              n190 = local read "Chirp Length (ms)"() -> (w374:i32)
              n191 = local read "Samples to Read"() -> (w370:i32)
              n192 = local read "Iterations"() -> (w367:i32)
              n193 = local read "Amplitude"() -> (w375:dbl)
              n194 = Number To Fractional String(number=w370, precision (6)=i16 3) -> (F-format string=w393:string)  [unwired: 2 in]
              n195 = Number To Fractional String(number=w367, precision (6)=i16 3) -> (F-format string=w368:string)  [unwired: 2 in]
              n196 = Number To Fractional String(number=w372, precision (6)=i16 3) -> (F-format string=w395:string)  [unwired: 2 in]
              n197 = Number To Fractional String(number=w375, precision (6)=i16 3) -> (F-format string=w403:string)  [unwired: 2 in]
              n198 = Number To Fractional String(number=w374, precision (6)=i16 3) -> (F-format string=w397:string)  [unwired: 2 in]
              n199 = Number To Fractional String(number=w373, precision (6)=i16 3) -> (F-format string=w396:string)  [unwired: 2 in]
              n200 = Number To Fractional String(number=w371, precision (6)=i16 3) -> (F-format string=w394:string)  [unwired: 2 in]
              n201 = Concatenate Strings("2. Length (ms): " ("string"), w397) -> (w384:string)
              n202 = Concatenate Strings("1. Amplitude (V): " ("string"), w403) -> (w385:string)
              n203 = Concatenate Strings("7. # of Iterations: " ("string"), w368) -> (w365:string)
              n204 = Concatenate Strings("6. #Samples to Read: " ("string"), w393) -> (w380:string)
              n205 = Concatenate Strings("3. Freq_Initial (Hz): " ("string"), w396) -> (w383:string)
              n206 = Concatenate Strings("4. Freq_Final (Hz): " ("string"), w395) -> (w382:string)
              n207 = Concatenate Strings("5. Interpulse Time (ms): " ("string"), w394) -> (w381:string)
              n208 = for {
                N: 7 -> [_]
                tunnel: w385 -> [w417]
                tunnel: w384 -> [w416]
                tunnel: w383 -> [w415]
                tunnel: w382 -> [w414]
                tunnel: w381 -> [w413]
                tunnel: w380 -> [w407]
                tunnel: w379 -> [w411]
                tunnel: w378 -> [w410]
                tunnel: [w409] -> w377
                tunnel: [w408] -> w376
                tunnel: w365 -> [w406]
                i -> [w412]
                n209 = Build Array(w417, w416, w415, w414, w413, w407, w406) -> (w420:string[])
                n210 = Index String Array(1:w412, 2:w420) -> (0:w419:string)  [unwired: 1 in]
                n211 = VISA Write(VISA resource name=w411, write buffer=w419, error in (no error)=w410) -> (VISA resource name out=w409:refnum<visa-resource-name>, error out=w408:errorcluster)  [unwired: 1 out]
                n212 = Wait (ms)(milliseconds to wait=u32 10) -> ()  [unwired: 1 out]
              }
            }
            frame "", Default {
            }
          }
        }
      }
    }
    n213 = Or(x=w30, y="?") -> (x .or. y?=w39:bool)
  }
  n214 = VISA Close(VISA resource name=w14, error in (no error)=w13) -> ()  [unwired: 1 out]
